vi "MinerJobDone.vi"(1 "chipID":string="2.4", 2 "RIG_IDENTIFIER":string="2.4", 3 "hashrate":dbl, 4 "duco_numeric_result":i32) -> (0 "concatenated string":string)   [LabVIEW 2014]
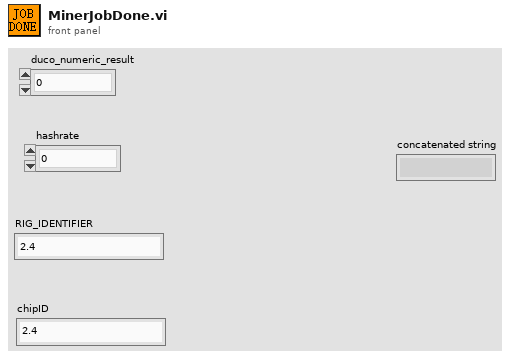
[diagram p1: front panel]
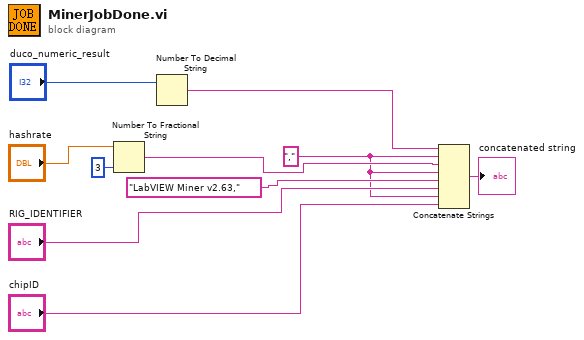
[diagram p0: block diagram]
diagram:
  w3 = "," ("string")
  n1 = Number To Fractional String(number="hashrate", precision (6)=i16 3) -> (F-format string=w6:string)  [unwired: 2 in]
  n2 = Number To Decimal String(number="duco_numeric_result") -> (decimal integer string=w9:string)  [unwired: 1 in]
  n3 = Concatenate Strings(w9, w3, w6, w3, "LabVIEW Miner v2.63," ("string"), "RIG_IDENTIFIER", w3, "chipID") -> (→"concatenated string":string)
